vi "Path to THIRD_PARTY_LICENSES--constant.vi"() -> (3 "appended path":path)   [LabVIEW 2025]
doc: "Represents the path to the THIRD_PARTY_LICENSES file.\n\nNote: this is necessary because the env-toolkit.vi will reside in G CLI Tools."
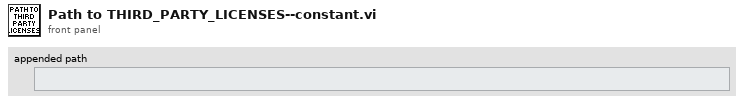
[diagram p1: front panel]
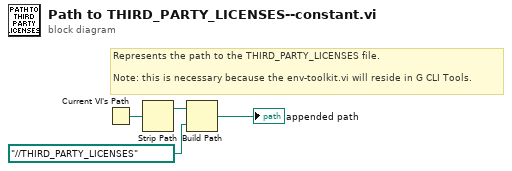
[diagram p0: block diagram]
diagram:
  # "Represents the path to the THIRD_PARTY_LICENSES file.\n\nNote: this is necessary because the env-toolkit.vi will reside in G CLI Tools."
  n1 = Current VI's Path() -> (path=w2:path)
  n2 = Strip Path(path=w2) -> (stripped path=w1:path)  [unwired: 1 out]
  n3 = Build Path(base path=w1, name or relative path=path "../../THIRD_PARTY_LICENSES") -> (appended path=→"appended path":path)
